vi "DriveEncReset.vi"(11 "DriveEnc?":bool) -> ()   [LabVIEW 2017]
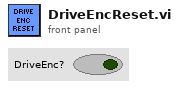
[diagram p1: front panel]
types:
  T1 = typedef "WPI_EncoderDevRef.ctl" = cluster{"DevStatus":errorcluster, "EncoderIndex":T2, "CounterIndex":T3, "DistancePerCount":dbl, "Decoding Type":T4}
  T2 = typedef "FPGA_EncoderIdx.ctl" = enum8{"Enc 0", "Enc 1", "Enc 2", "Enc 3", "Enc 4", "Enc 5", "Enc 6", "Enc 7", "Invalid"}
  T3 = typedef "FPGA_CounterCtrSystemIndex.ctl" = enum8{"Ctr 0", "Ctr 1", "Ctr 2", "Ctr 3", "Ctr 4", "Ctr 5", "Ctr 6", "Ctr 7", "Invalid"}
  T4 = typedef "WPI_EncoderType.ctl" = enum16{"1x", "2x", "4x"}
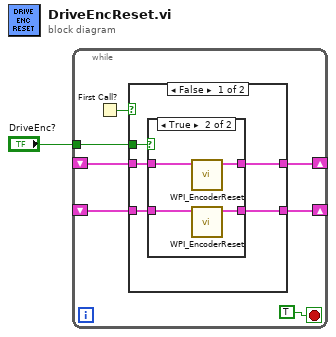
[diagram p0: block diagram]
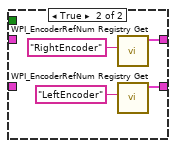
[diagram p3: hidden frame]
diagram:
  n1 = while {
    tunnel: "DriveEnc?" -> [w8]
    shift-right: [w6] -> _
    shift-left: _ -> [w4]
    shift-right: [w7] -> _
    shift-left: _ -> [w5]
    stop <- TRUE stop-if-true
    n2 = First Call?() -> (First Call?: T/F=w3:bool)
    n3 = case shown="False" w3 {
      tunnel: w8 -> [w13 _]
      tunnel: [w11 w21] -> w6
      tunnel: [w9 w20] -> w7
      tunnel: w5 -> [w10 _]
      tunnel: w4 -> [w12 _]
      frame False {
        n4 = case shown="True" w13 {
          tunnel: [w15 w16] -> w11
          tunnel: w12 -> [w15 w17]
          tunnel: [w14 w18] -> w9
          tunnel: w10 -> [w14 w19]
          frame False {
          }
          frame True {
            n5 = call <vilib>:"WPI_EncoderReset.vi"("EncoderDevRef"=w19) -> ("EncoderDevRef"=w18:T1)  [unwired: 9 in, 1 out]
            n6 = call <vilib>:"WPI_EncoderReset.vi"("EncoderDevRef"=w17) -> ("EncoderDevRef"=w16:T1)  [unwired: 9 in, 1 out]
          }
        }
      }
      frame True {
        n7 = call <vilib>:"WPI_EncoderRefNum Registry Get.vi"("refnum name"="RightEncoder") -> ("EncoderDevRef"=w20:T1)  [unwired: 9 in, 1 out]
        n8 = call <vilib>:"WPI_EncoderRefNum Registry Get.vi"("refnum name"="LeftEncoder") -> ("EncoderDevRef"=w21:T1)  [unwired: 9 in, 1 out]
      }
    }
  }
